vi "Create Sessions Impl.vi"(7 "require single session":bool, 8 "error in":errorcluster, 10 "instrument":refnum<class "IInstrument.lvclass">, 11 "session reservation in":refnum<class "Session Reservation.lvclass">) -> (0 "error out":errorcluster, 1 "channel lists":string[](array[string]), 2 "sessions":variant[](array[variant]), 3 "session reservation out":refnum<class "Session Reservation.lvclass">)   [LabVIEW 2020, in "MeasurementLink Session Management.lvlib" / "Session Reservation.lvclass"]
uses:
  Session Reservation.lvclass
  MeasurementLink Instrument/IInstrument/IInstrument.lvclass
  Session Reservation.lvclass/Session Reservation.ctl
  MeasurementLink Instrument/IInstrument/Initialize Session Behavior.ctl
  MeasurementLink Instrument/IInstrument/Close Session Behavior.ctl
  MeasurementLink gRPC Utilities/Service Location FGV.vi
  MeasurementLink Measurement Server/Helpers/Error Strings Global Internal.vi
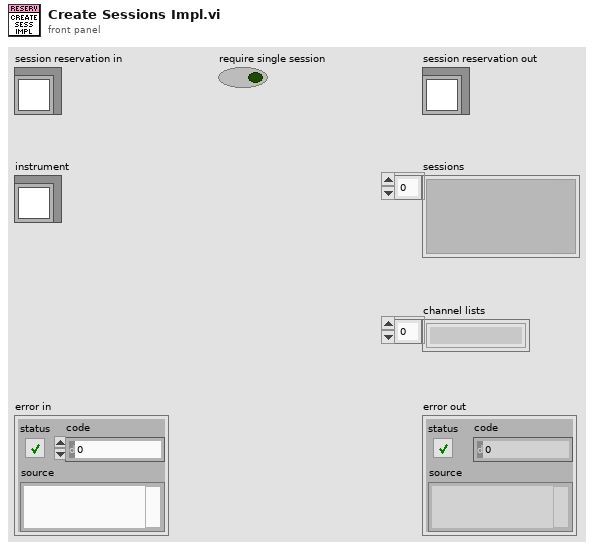
[diagram p1: front panel]
types:
  T1 = typedef "MeasurementLink Instrument.lvlib/IInstrument.lvclass/Close Session Behavior.ctl" = enum16{"Close Session", "Detach Session"}
  T2 = typedef "MeasurementLink Instrument.lvlib/IInstrument.lvclass/Initialize Session Behavior.ctl" = enum16{"Create Session", "Attach Session"}
  T3 = typedef "MeasurementLink Session Management.lvlib/Session Reservation.lvclass/Data.ctl" = cluster{"session and driver infos":T4[]}
  T4 = typedef "MeasurementLink Session Management.lvlib/Session Reservation.lvclass/Session and Driver Info.ctl" = cluster{"session info":T5, "session":variant}
  T5 = typedef "MeasurementLink Session Management Client.lvlib/ni_measurementlink_sessionmanagement_v1_SessionInformation.ctl" = cluster{"session":T6, "resource_name":string, "channel_list":string, "instrument_type_id":string, "session_exists":bool, "channel_mappings":T7[]}
  T6 = typedef "MeasurementLink Session Management Client.lvlib/nidevice_grpc_Session.ctl" = cluster{"name":string}
  T7 = typedef "MeasurementLink Session Management Client.lvlib/ni_measurementlink_sessionmanagement_v1_ChannelMapping.ctl" = cluster{"pin_or_relay_name":string, "site":i32, "channel":string}
  T8 = typedef "MeasurementLink Instrument.lvlib/IInstrument.lvclass/Remote Connection Options.ctl" = cluster{"session name":string, "address":string, "port":u32}
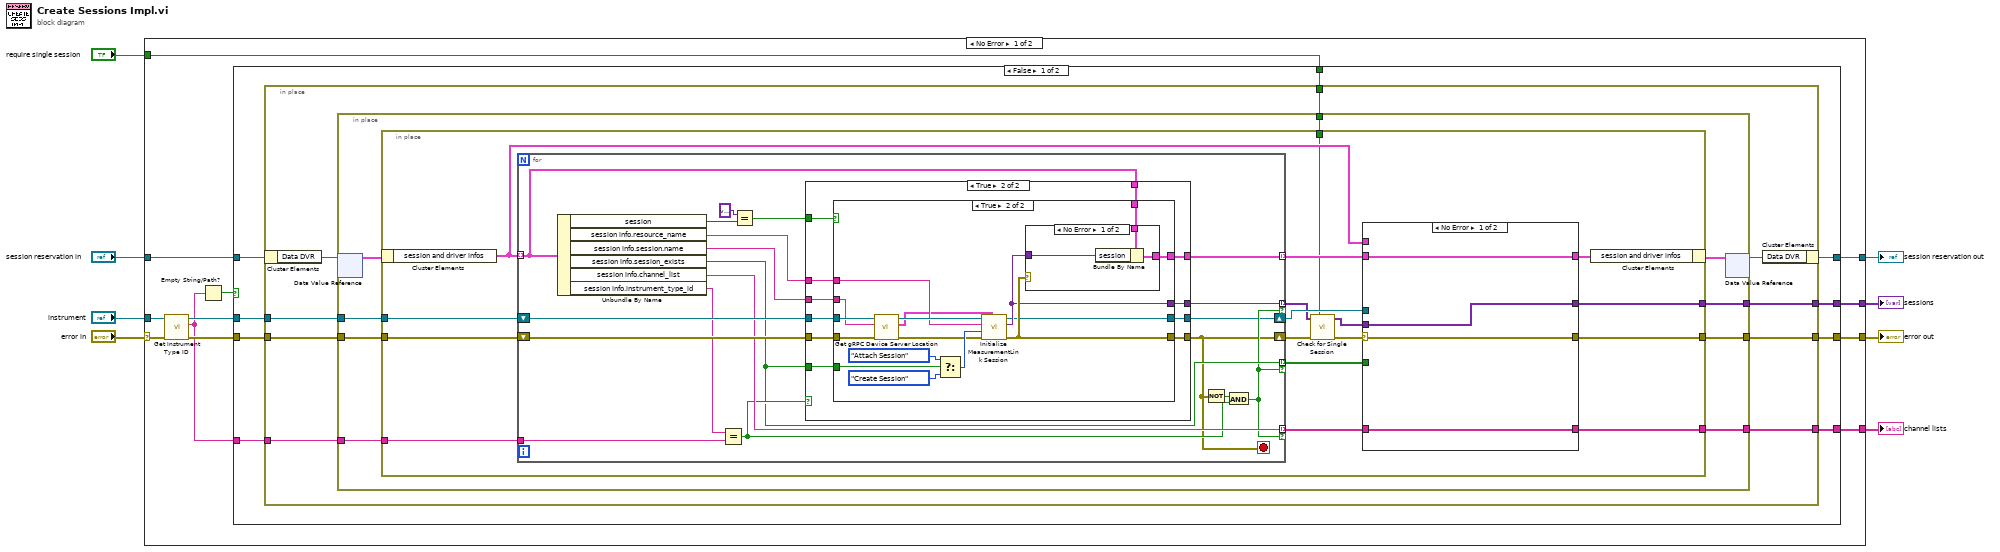
[diagram p0: block diagram]
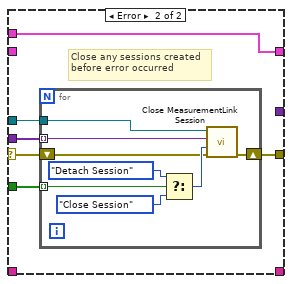
[diagram p2: hidden frame]
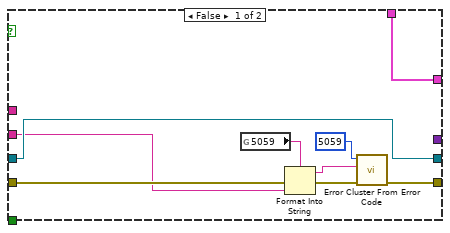
[diagram p4: hidden frame]
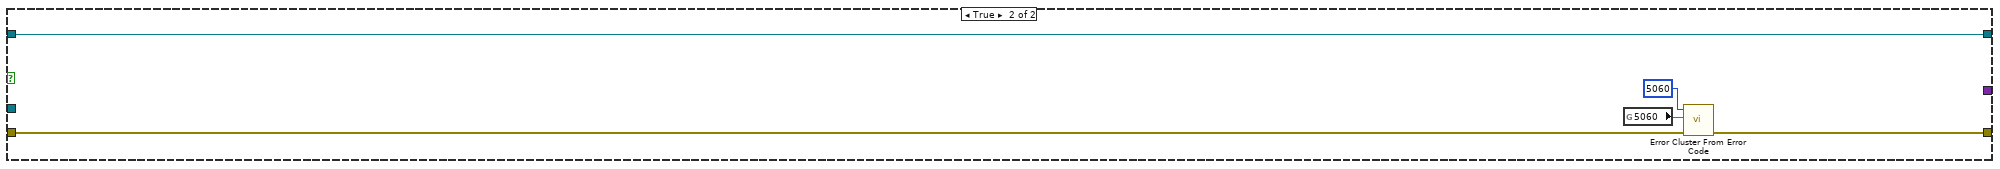
[diagram p6: hidden frame]
diagram:
  n1 = case shown="No Error" "error in" {
    selector: "error in" -> [w15 w151]
    tunnel: "session reservation in" -> [w20 w150]
    tunnel: "instrument" -> [w14 _]
    tunnel: [w19 _] -> w5
    tunnel: [w18 w151] -> w4
    tunnel: [w17 _] -> w3
    tunnel: [w16 w150] -> w2
    tunnel: "require single session" -> [w11 _]
    frame No Error {
      n2 = call-dynamic "Get Instrument Type ID.vi"("error in (no error)"=w15, "instrument in"=w14) -> ("error out"=w12:errorcluster, "instrument type id"=w9:string, "instrument out"=w13:refnum<class "IInstrument.lvclass">)  [unwired: 7 in]
      n3 = Empty String/Path?(string/path=w9) -> (empty?=w10:bool)
      n4 = case shown="False" w10 {
        tunnel: w20 -> [w29 w149]
        tunnel: [w28 _] -> w19
        tunnel: [w27 w146] -> w18
        tunnel: [w26 _] -> w17
        tunnel: [w25 w149] -> w16
        tunnel: w9 -> [w24 _]
        tunnel: w13 -> [w23 _]
        tunnel: w12 -> [w22 w145]
        tunnel: w11 -> [w21 _]
        frame False {
          n5 = in-place {
            in-place-border: [w36] -> w28
            in-place-border: [w35] -> w27
            in-place-border: [w34] -> w26
            in-place-border: w24 -> [w33]
            in-place-border: w23 -> [w32]
            in-place-border: w22 -> [w31]
            in-place-border: w21 -> [w30]
            n6 = in-place-cluster #1(w29) -> ("Data DVR"=w38:refnum<data-value>)
            n7 = in-place {
              in-place-border: [w47] -> w36
              in-place-border: [w46] -> w35
              in-place-border: [w45] -> w34
              in-place-border: w33 -> [w44]
              in-place-border: w32 -> [w43]
              in-place-border: w31 -> [w42]
              in-place-border: w30 -> [w39]
              n8 = in-place-dvr #2(w38) -> (w41:T3)  [unwired: 1 out]
              n9 = in-place {
                in-place-border: [w60] -> w47
                in-place-border: [w61] -> w46
                in-place-border: [w56] -> w45
                in-place-border: w44 -> [w64]
                in-place-border: w43 -> [w63]
                in-place-border: w42 -> [w62]
                in-place-border: w39 -> [w48]
                n10 = in-place-cluster #3(w41) -> ("session and driver infos"=w55:T4[])
                n11 = for {
                  tunnel: w55 -> [w99] mode=indexing
                  tunnel: [w100] -> w50 mode=indexing if=w85
                  shift-right: [w83] -> w52
                  shift-left: w62 -> [w95]
                  tunnel: [w92] -> w57 mode=indexing if=w85
                  tunnel: [w98] -> w59 mode=indexing
                  tunnel: w64 -> [w97]
                  tunnel: [w86] -> w54 mode=indexing if=w85
                  shift-right: [w84] -> w53
                  shift-left: w63 -> [w96]
                  stop <- w83 stop-if-true
                  n12 = Unbundle By Name(w99) -> ("session"=w91:variant, "session info.resource_name"=w93:string, "session info.session.name"=w101:string, "session info.session_exists"=w86:bool, "session info.channel_list"=w92:string, "session info.instrument_type_id"=w94:string)
                  n13 = Equal?(x=w94, y=w97) -> (x = y?=w87:bool)
                  n14 = Equal?(x=variant, y=w91) -> (x = y?=w90:bool)
                  n15 = case shown="True" w87 {
                    tunnel: w101 -> [_ w115]
                    tunnel: [_ w111] -> w100
                    tunnel: w93 -> [_ w114]
                    tunnel: w86 -> [_ w113]
                    tunnel: [w103 w112] -> w83
                    tunnel: w99 -> [w104 w110]
                    tunnel: [w104 w109] -> w98
                    tunnel: w96 -> [w102 w108]
                    tunnel: w95 -> [w103 w107]
                    tunnel: w90 -> [_ w106]
                    tunnel: [w102 w105] -> w84
                    frame False {
                    }
                    frame True {
                      n16 = case shown="True" w106 {
                        tunnel: w115 -> [w116 w127]
                        tunnel: w114 -> [_ w126]
                        tunnel: w113 -> [_ w138]
                        tunnel: [w123 w136] -> w112
                        tunnel: [_ w135] -> w111
                        tunnel: w110 -> [w122 w134]
                        tunnel: [w122 w133] -> w109
                        tunnel: w108 -> [w117 w131]
                        tunnel: w107 -> [w121 w129]
                        tunnel: [w117 w132] -> w105
                        frame False {
                          n17 = global read "Error Strings Global Internal.vi" "5059"() -> (w118:string)
                          n18 = Format Into String(format string=w118, error in=w121, w116) -> (resulting string=w119:string, error out=w120:errorcluster)  [unwired: 1 in]
                          n19 = call <vilib>:"Error Cluster From Error Code.vi"("error in (no error)"=w120, "error message (\"\")"=w119, "error code (0)"=5059) -> ("error out"=w123:errorcluster)  [unwired: 6 in]
                        }
                        frame True {
                          n20 = call "Get gRPC Device Server Location.vi"("error in"=w129, "session name"=w127, "instrument in"=w131) -> ("error out"=w128:errorcluster, "remote connection options"=w125:T8, "instrument out"=w130:refnum<class "IInstrument.lvclass">)  [unwired: 6 in]
                          n21 = Select(t=Initialize_Session_Behavior."Attach Session", s=w138, f=Initialize_Session_Behavior."Create Session" ("initialize session behavior")) -> (s? t:f=w137:T2)
                          n22 = call-dynamic "Initialize MeasurementLink Session.vi"("remote connection options"=w125, "error in (no error)"=w128, "initialize session behavior"=w137, "resource name"=w126, "instrument in"=w130) -> ("error out"=w136:errorcluster, "session out"=w135:variant, "instrument out"=w132:refnum<class "IInstrument.lvclass">)  [unwired: 4 in]
                          n23 = case shown="No Error" w136 {
                            tunnel: w135 -> [w143 _]
                            tunnel: w134 -> [w142 w144]
                            tunnel: [w141 w144] -> w133
                            frame No Error {
                              n24 = Bundle By Name(cluster=w142, "session"=w143) -> (w141:T4)
                            }
                            frame Error {
                            }
                          }
                        }
                      }
                    }
                  }
                  n25 = Not(x=w83) -> (.not. x?=w88:bool)
                  n26 = And(x=w88, y=w87) -> (x .and. y?=w85:bool)
                }
                n27 = call "Check for Single Session.vi"("perform check"=w48, "error in"=w52, "sessions in"=w50) -> ("error out"=w51:errorcluster, "sessions out"=w49:variant[])  [unwired: 7 in]
                n28 = case shown="No Error" w51 {
                  selector: w51 -> [w68 w69]
                  tunnel: [w68 w73] -> w61
                  tunnel: w49 -> [w67 w71]
                  tunnel: [w67 _] -> w60
                  tunnel: w59 -> [w66 _]
                  tunnel: [w66 w74] -> w58
                  tunnel: w57 -> [w65 _]
                  tunnel: [w65 _] -> w56
                  tunnel: w55 -> [_ w74]
                  tunnel: w54 -> [_ w70]
                  tunnel: w53 -> [_ w72]
                  frame No Error {
                  }
                  frame Error {
                    # "Close any sessions created\nbefore error occurred"
                    n29 = for {
                      tunnel: w72 -> [w81]
                      tunnel: w71 -> [w80] mode=indexing
                      tunnel: w70 -> [w76] mode=indexing
                      shift-right: [w82] -> w73
                      shift-left: w69 -> [w75]
                      n30 = Select(t=Close_Session_Behavior."Detach Session" ("close session behavior"), s=w76, f=Close_Session_Behavior."Close Session") -> (s? t:f=w79:T1)
                      n31 = call-dynamic "Close MeasurementLink Session.vi"("error in (no error)"=w75, "close session behavior"=w79, "session in"=w80, "instrument in"=w81) -> ("error out"=w82:errorcluster)  [unwired: 7 in]
                    }
                  }
                }
                n32 = in-place-cluster #3("session and driver infos"=w58) -> (w40:T3)
              }
              n33 = in-place-dvr #2(w40) -> (w37:refnum<data-value>)  [unwired: 1 out]
            }
            n34 = in-place-cluster #1("Data DVR"=w37) -> (w25:refnum<class "Session Reservation.lvclass">)
          }
        }
        frame True {
          n35 = global read "Error Strings Global Internal.vi" "5060"() -> (w147:string)
          n36 = call <vilib>:"Error Cluster From Error Code.vi"("error in (no error)"=w145, "error message (\"\")"=w147, "error code (0)"=5060) -> ("error out"=w146:errorcluster)  [unwired: 6 in]
        }
      }
    }
    frame Error {
    }
  }
  "error out" <- w4
  "sessions" <- w5
  "session reservation out" <- w2
  "channel lists" <- w3
